vi "Set Routing Channel Initial State.vi"(8 "error in (no error)":errorcluster, 10 "State":string, 11 "Channel Ref in":T1 format="%.0x") -> (0 "error out":errorcluster, 3 "Channel Ref out":T1=18446744073709551615 format="%.0x")   [LabVIEW 2017, in "Routing and Faulting Scripting.lvlib"]
uses:
  Routing and Faulting Scripting.lvlib
  <vilib>/NI Veristand/Custom Device API/Custom Device Item Ref.ctl
  <vilib>/NI VeriStand/Custom Device API/Custom Device API.lvlib
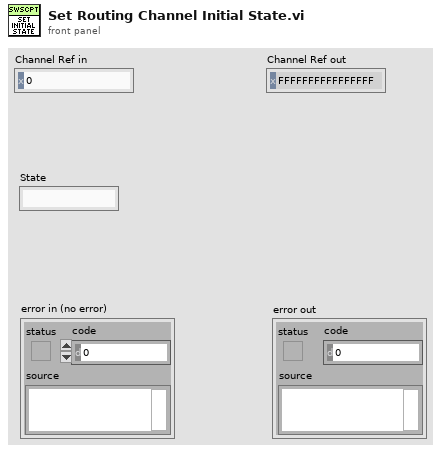
[diagram p1: front panel]
types:
  T1 = typedef "Custom Device API.lvlib/Custom Device Item Ref.ctl" = u64
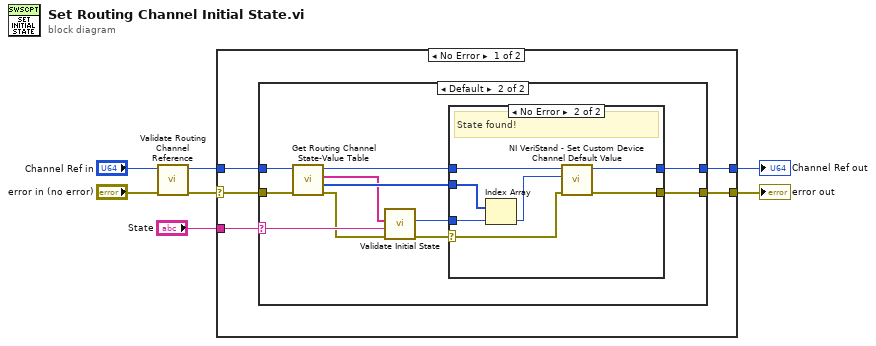
[diagram p0: block diagram]
diagram:
  n1 = call "Validate Routing Channel Reference.vi"("error in (no error)"="error in (no error)", "Channel Ref in"="Channel Ref in") -> ("error out"=w3:errorcluster, "Channel Ref out"=w1:T1)  [unwired: 8 in]
  n2 = case shown="No Error" w3 {
    selector: w3 -> [w11 w36]
    tunnel: [w9 w36] -> w4
    tunnel: w1 -> [w12 w35]
    tunnel: [w10 w35] -> w6
    tunnel: "State" -> [w8 _]
    frame No Error {
      n3 = case shown="Default" w8 {
        selector: w8 -> [_ w18]
        tunnel: w12 -> [w13 w25]
        tunnel: w11 -> [w14 w24]
        tunnel: [w13 w21] -> w10
        tunnel: [w14 w20] -> w9
        frame "" {
        }
        frame Default {
          n4 = call "Get Routing Channel State-Value Table.vi"("error in (no error)"=w24, "Channel Ref in"=w25) -> ("error out"=w17:errorcluster, "State Values"=w22:i32[], "State Names"=w19:string[], "Channel Ref out"=w23:T1)  [unwired: 6 in]
          n5 = call "Validate Initial State.vi"("error in (no error)"=w17, "Intial State"=w18, "State Names"=w19) -> ("error out"=w16:errorcluster, "index found"=w15:i32)  [unwired: 7 in]
          n6 = case shown="No Error" w16 {
            selector: w16 -> [w26 w29]
            tunnel: w23 -> [w27 w34]
            tunnel: w22 -> [_ w33]
            tunnel: [w27 w31] -> w21
            tunnel: [w26 w30] -> w20
            tunnel: w15 -> [_ w28]
            frame Error {
              # "State not found"
            }
            frame No Error {
              # "State found!"
              n7 = Index Array(array=w33, index=w28) -> (element=w32:i32)
              n8 = call <vilib>:"NI VeriStand - Set Custom Device Channel Default Value.vi"("error in (no error)"=w29, "Default Value"=w32, "Channel Ref in"=w34) -> ("error out"=w30:errorcluster, "Channel Ref out"=w31:T1)  [unwired: 7 in]
            }
          }
        }
      }
    }
    frame Error {
    }
  }
  "Channel Ref out" <- w6
  "error out" <- w4
